vi "Configure Units.vi"(8 "error in (no error)":errorcluster, 10 "Units (0: Gram)":u16(ring) items=["Gram (g)"=0, "Kilogram (kg)"=1, "Penny weight (dwt)"=2, "Carat (ct)"=3, "Ounce (oz)"=4, "Ounce Troy (oz t)"=5, "Grain (GN)"=6, "Hong Kong Tael (HKt)"=7, "Singapore Tael (SGt)"=8, "Tiwan Tael (TWt)"=9, "Momme (m)"=10, "Pound (lb)"=11, "Newton (N)"=13, "Tical (ti)"=14, "Tula"=15, "Mesghal (Meshg)"=16, "Baht"=17, "Custom"=19], 11 "VISA resource name":refnum<visa-resource-name>) -> (0 "error out":errorcluster, 3 "VISA resource name out":refnum<visa-resource-name>)   [LabVIEW 2015, in "Ohaus AV Series.lvlib"]
doc: "This VI changes the units to perform measurements in.\n\nNote:\n\n(1) The Unit of choice must be enabled in the balances menu before being selected.\n\nThese settings are under:\n\nMenu\n Unit\n [Unit of Interest]\n Set On"
uses:
  Ohaus AV Series.lvlib
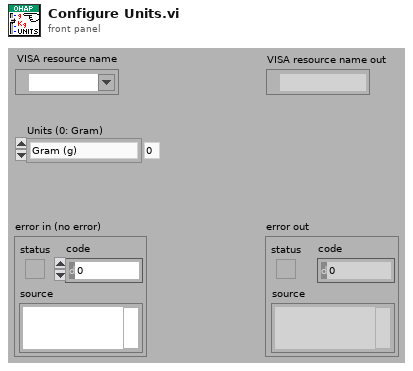
[diagram p1: front panel]
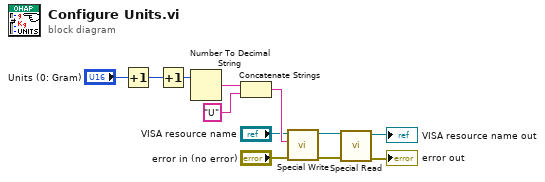
[diagram p0: block diagram]
diagram:
  n1 = Increment(x="Units (0: Gram)") -> (x+1=w6:u16)
  n2 = Increment(x=w6) -> (x+1=w5:u16)
  n3 = Number To Decimal String(number=w5) -> (decimal integer string=w9:string)  [unwired: 1 in]
  n4 = Concatenate Strings(w9, "U" ("string")) -> (w7:string)
  n5 = call "Special Write.vi"("error in (no error)"="error in (no error)", "Input String"=w7, "VISA resource name"="VISA resource name") -> ("error out"=w10:errorcluster, "VISA resource name out"=w11:refnum<visa-resource-name>)  [unwired: 7 in]
  n6 = call "Special Read.vi"("error in (no error)"=w10, "VISA resource name"=w11) -> ("error out"=→"error out":errorcluster, "VISA resource name out"=→"VISA resource name out":refnum<visa-resource-name>)  [unwired: 7 in, 1 out]
